vi "Dispose.vi"(0 "object in":refnum<class "EmergencyController.lvclass">, 5 "error in (no error)":errorcluster) -> (14 "object out":refnum<class "EmergencyController.lvclass">, 19 "error out":errorcluster)   [LabVIEW 2014, in "EmergencyController.lvclass"]
uses:
  EmergencyController.lvclass
  EmergencyController.lvclass/EmergencyController.ctl
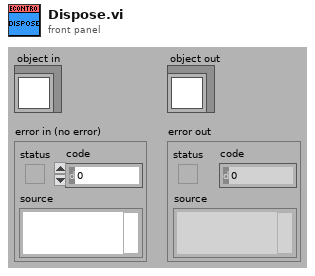
[diagram p1: front panel]
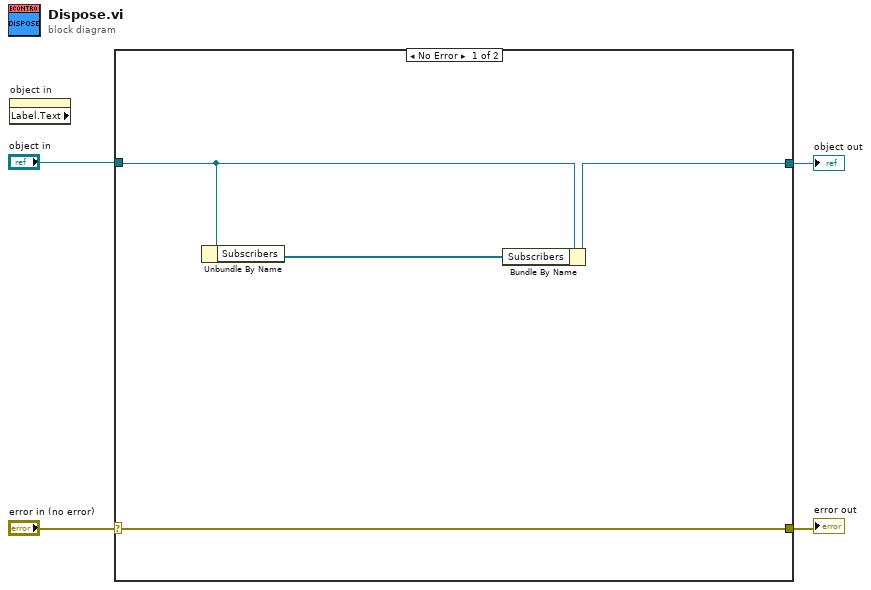
[diagram p0: block diagram]
diagram:
  n1 = property on="object in" class="LVClassControl (strict)" props=["Label", "Text"]() -> ()  [unwired: 2 in, 3 out]
  n2 = case shown="No Error" "error in (no error)" {
    selector: "error in (no error)" -> [w7 w10]
    tunnel: [w7 w10] -> w3
    tunnel: [w5 w9] -> w1
    tunnel: "object in" -> [w6 w9]
    frame No Error {
      n3 = Unbundle By Name(w6) -> ("Subscribers"=w8:refnum<class>[])
      n4 = Bundle By Name(cluster=w6, "Subscribers"=w8) -> (w5:refnum<class "EmergencyController.lvclass">)
    }
    frame Error {
    }
  }
  "error out" <- w3
  "object out" <- w1
